vi "AutoRoutineSelector.vi"(6 "NotPurePursuit":bool, 8 "Routine":T1, 9 "OurSwitch":bool, 10 "OurScale":bool, 11 "Position":dbl) -> (3 "File Name":string)   [LabVIEW 2017]
uses:
  Shared/AutoRoutineSelector.ctl
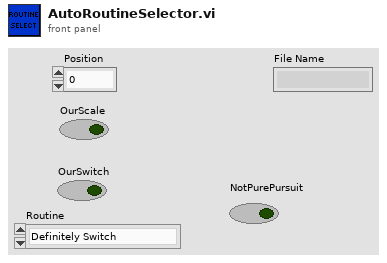
[diagram p1: front panel]
types:
  T1 = typedef "AutoRoutineSelector.ctl" = enum16{"Definitely Switch", "Definitely Scale", "Switch if in front, else scale", "Scale if in front, else switch", "Switch if in front, else cross line", "Scale if in front, else cross line", "Switch if in front, else scale if in front, else cross line ", "Scale if in front, else switch if in front, else cross line ", "Drive across line"}
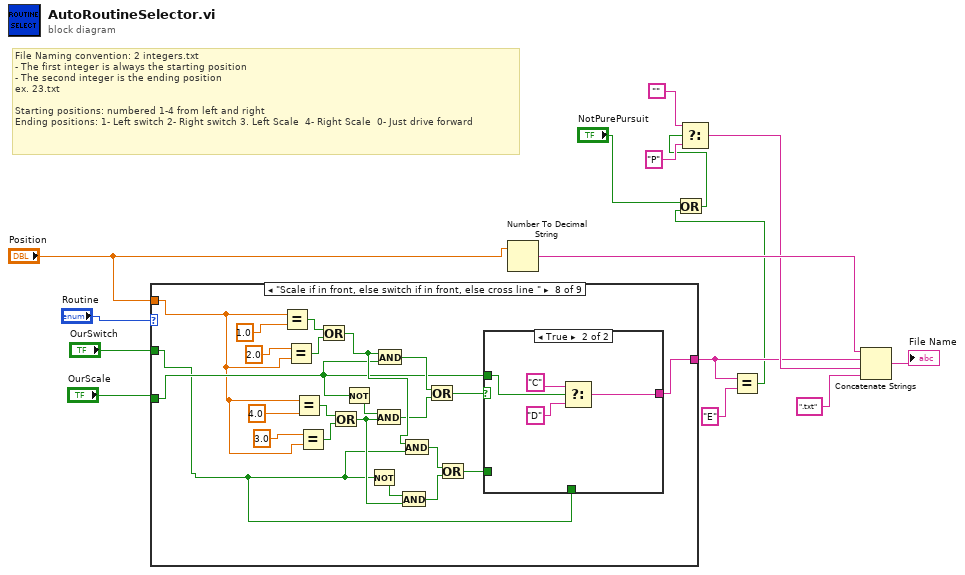
[diagram p0: block diagram]
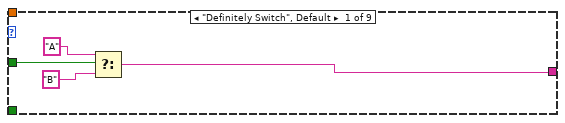
[diagram p2: hidden frame]
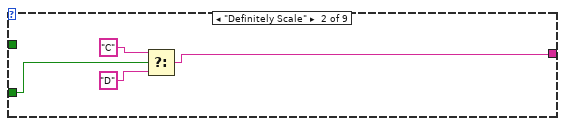
[diagram p3: hidden frame]
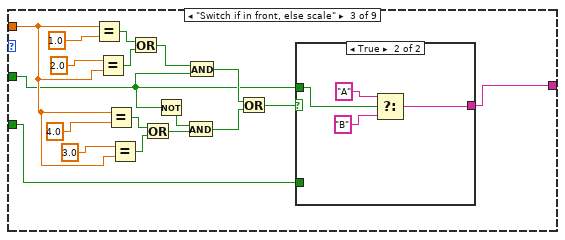
[diagram p4: hidden frame]
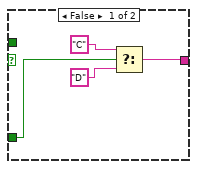
[diagram p5: hidden frame]
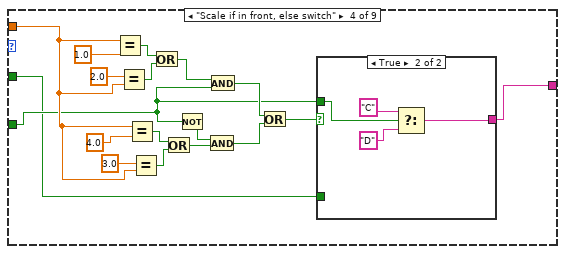
[diagram p6: hidden frame]
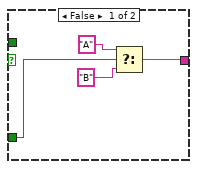
[diagram p7: hidden frame]
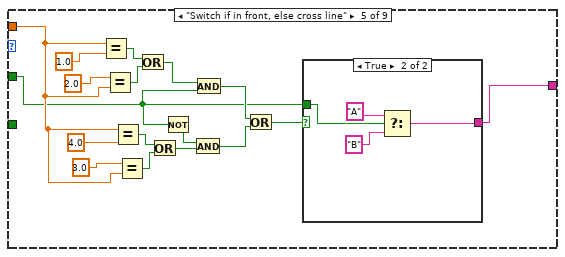
[diagram p8: hidden frame]
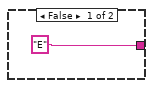
[diagram p9: hidden frame]
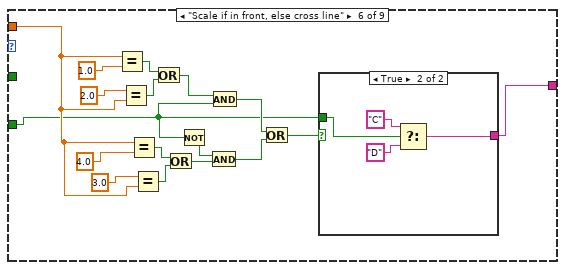
[diagram p10: hidden frame]
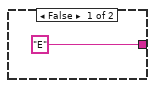
[diagram p11: hidden frame]
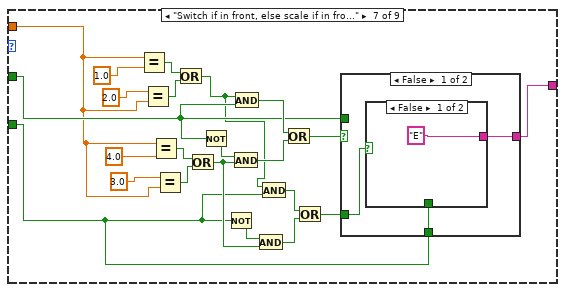
[diagram p12: hidden frame]
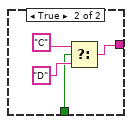
[diagram p13: hidden frame]
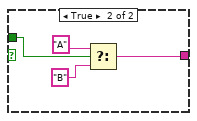
[diagram p14: hidden frame]
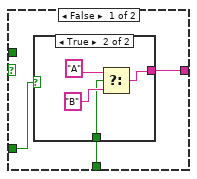
[diagram p15: hidden frame]
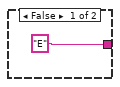
[diagram p16: hidden frame]
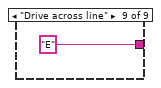
[diagram p17: hidden frame]
diagram:
  # "File Naming convention: 2 integers.txt \n- The first integer is always the starting position\n- The second integer is the ending position\nex. 23.txt\n\nStarting positions: numbered 1-4 from left and right\nEnding positions: 1- Left switch 2- Right switch 3. Left Scale  4- Right Scale  0- Just drive forward"
  n1 = case shown="\"Scale if in front, else switch if in front, else cross line \"" "Routine" {
    tunnel: "OurSwitch" -> [w19 _ w30 w55 w81 _ w129 w156 _]
    tunnel: "OurScale" -> [_ w23 w29 w56 _ w103 w120 w157 _]
    tunnel: [w16 w20 w24 w50 w76 w98 w127 w154 "E"] -> w4
    tunnel: "Position" -> [_ _ w36 w57 w82 w104 w128 w155 _]
    frame "Definitely Switch", Default {
      n2 = Select(t="A", s=w19, f="B") -> (s? t:f=w16:string)
    }
    frame "Definitely Scale" {
      n3 = Select(t="C", s=w23, f="D") -> (s? t:f=w20:string)
    }
    frame "Switch if in front, else scale" {
      n4 = Equal?(x=w36, y=1.0) -> (x = y?=w41:bool)
      n5 = Equal?(x=2.0 ("y"), y=w36) -> (x = y?=w40:bool)
      n6 = Equal?(x=w36, y=4.0) -> (x = y?=w37:bool)
      n7 = Equal?(x=3.0 ("y"), y=w36) -> (x = y?=w38:bool)
      n8 = Or(x=w41, y=w40) -> (x .or. y?=w39:bool)
      n9 = Or(x=w37, y=w38) -> (x .or. y?=w35:bool)
      n10 = Not(x=w30) -> (.not. x?=w34:bool)
      n11 = And(x=w34, y=w35) -> (x .and. y?=w32:bool)
      n12 = And(x=w39, y=w30) -> (x .and. y?=w33:bool)
      n13 = Or(x=w33, y=w32) -> (x .or. y?=w31:bool)
      n14 = case shown="True" w31 {
        tunnel: w30 -> [_ w49]
        tunnel: [w44 w46] -> w24
        tunnel: w29 -> [w45 _]
        frame False {
          n15 = Select(t="C", s=w45, f="D") -> (s? t:f=w44:string)
        }
        frame True {
          n16 = Select(t="A", s=w49, f="B") -> (s? t:f=w46:string)
        }
      }
    }
    frame "Scale if in front, else switch" {
      n17 = Equal?(x=w57, y=1.0) -> (x = y?=w58:bool)
      n18 = Equal?(x=2.0 ("y"), y=w57) -> (x = y?=w59:bool)
      n19 = Equal?(x=w57, y=4.0) -> (x = y?=w62:bool)
      n20 = Equal?(x=3.0 ("y"), y=w57) -> (x = y?=w61:bool)
      n21 = Or(x=w58, y=w59) -> (x .or. y?=w60:bool)
      n22 = Or(x=w62, y=w61) -> (x .or. y?=w63:bool)
      n23 = Not(x=w56) -> (.not. x?=w64:bool)
      n24 = And(x=w64, y=w63) -> (x .and. y?=w66:bool)
      n25 = And(x=w60, y=w56) -> (x .and. y?=w65:bool)
      n26 = Or(x=w65, y=w66) -> (x .or. y?=w67:bool)
      n27 = case shown="True" w67 {
        tunnel: w56 -> [_ w75]
        tunnel: [w70 w72] -> w50
        tunnel: w55 -> [w71 _]
        frame False {
          n28 = Select(t="A", s=w71, f="B") -> (s? t:f=w70:string)
        }
        frame True {
          n29 = Select(t="C", s=w75, f="D") -> (s? t:f=w72:string)
        }
      }
    }
    frame "Switch if in front, else cross line" {
      n30 = Equal?(x=w82, y=1.0) -> (x = y?=w83:bool)
      n31 = Equal?(x=2.0 ("y"), y=w82) -> (x = y?=w84:bool)
      n32 = Equal?(x=w82, y=4.0) -> (x = y?=w87:bool)
      n33 = Equal?(x=3.0 ("y"), y=w82) -> (x = y?=w86:bool)
      n34 = Or(x=w83, y=w84) -> (x .or. y?=w85:bool)
      n35 = Or(x=w87, y=w86) -> (x .or. y?=w88:bool)
      n36 = Not(x=w81) -> (.not. x?=w89:bool)
      n37 = And(x=w89, y=w88) -> (x .and. y?=w91:bool)
      n38 = And(x=w85, y=w81) -> (x .and. y?=w90:bool)
      n39 = Or(x=w90, y=w91) -> (x .or. y?=w92:bool)
      n40 = case shown="True" w92 {
        tunnel: w81 -> [_ w97]
        tunnel: ["E" w94] -> w76
        frame False {
        }
        frame True {
          n41 = Select(t="A", s=w97, f="B") -> (s? t:f=w94:string)
        }
      }
    }
    frame "Scale if in front, else cross line" {
      n42 = Equal?(x=w104, y=1.0) -> (x = y?=w114:bool)
      n43 = Equal?(x=2.0 ("y"), y=w104) -> (x = y?=w113:bool)
      n44 = Equal?(x=w104, y=4.0) -> (x = y?=w110:bool)
      n45 = Equal?(x=3.0 ("y"), y=w104) -> (x = y?=w111:bool)
      n46 = Or(x=w114, y=w113) -> (x .or. y?=w112:bool)
      n47 = Or(x=w110, y=w111) -> (x .or. y?=w109:bool)
      n48 = Not(x=w103) -> (.not. x?=w108:bool)
      n49 = And(x=w108, y=w109) -> (x .and. y?=w106:bool)
      n50 = And(x=w112, y=w103) -> (x .and. y?=w107:bool)
      n51 = Or(x=w107, y=w106) -> (x .or. y?=w105:bool)
      n52 = case shown="True" w105 {
        tunnel: w103 -> [_ w119]
        tunnel: ["E" w116] -> w98
        frame False {
        }
        frame True {
          n53 = Select(t="C", s=w119, f="D") -> (s? t:f=w116:string)
        }
      }
    }
    frame "Switch if in front, else scale if in front, else cross line " {
      n54 = Equal?(x=w128, y=1.0) -> (x = y?=w141:bool)
      n55 = Equal?(x=2.0 ("y"), y=w128) -> (x = y?=w140:bool)
      n56 = Equal?(x=w128, y=4.0) -> (x = y?=w138:bool)
      n57 = Equal?(x=3.0 ("y"), y=w128) -> (x = y?=w139:bool)
      n58 = Or(x=w141, y=w140) -> (x .or. y?=w124:bool)
      n59 = Or(x=w138, y=w139) -> (x .or. y?=w125:bool)
      n60 = Not(x=w129) -> (.not. x?=w137:bool)
      n61 = Not(x=w120) -> (.not. x?=w126:bool)
      n62 = And(x=w137, y=w125) -> (x .and. y?=w135:bool)
      n63 = And(x=w124, y=w129) -> (x .and. y?=w136:bool)
      n64 = And(x=w126, y=w125) -> (x .and. y?=w122:bool)
      n65 = And(x=w124, y=w120) -> (x .and. y?=w123:bool)
      n66 = Or(x=w136, y=w135) -> (x .or. y?=w134:bool)
      n67 = Or(x=w123, y=w122) -> (x .or. y?=w121:bool)
      n68 = case shown="False" w134 {
        tunnel: w129 -> [_ w153]
        tunnel: [w144 w150] -> w127
        tunnel: w121 -> [w143 _]
        tunnel: w120 -> [w142 _]
        frame False {
          n69 = case shown="False" w143 {
            tunnel: ["E" w147] -> w144
            tunnel: w142 -> [_ w146]
            frame False {
            }
            frame True {
              n70 = Select(t="C", s=w146, f="D") -> (s? t:f=w147:string)
            }
          }
        }
        frame True {
          n71 = Select(t="A", s=w153, f="B") -> (s? t:f=w150:string)
        }
      }
    }
    frame "Scale if in front, else switch if in front, else cross line " {
      n72 = Equal?(x=w155, y=1.0) -> (x = y?=w162:bool)
      n73 = Equal?(x=2.0 ("y"), y=w155) -> (x = y?=w163:bool)
      n74 = Equal?(x=w155, y=4.0) -> (x = y?=w165:bool)
      n75 = Equal?(x=3.0 ("y"), y=w155) -> (x = y?=w164:bool)
      n76 = Or(x=w162, y=w163) -> (x .or. y?=w172:bool)
      n77 = Or(x=w165, y=w164) -> (x .or. y?=w171:bool)
      n78 = Not(x=w157) -> (.not. x?=w166:bool)
      n79 = Not(x=w156) -> (.not. x?=w170:bool)
      n80 = And(x=w166, y=w171) -> (x .and. y?=w168:bool)
      n81 = And(x=w172, y=w157) -> (x .and. y?=w167:bool)
      n82 = And(x=w170, y=w171) -> (x .and. y?=w174:bool)
      n83 = And(x=w172, y=w156) -> (x .and. y?=w173:bool)
      n84 = Or(x=w167, y=w168) -> (x .or. y?=w169:bool)
      n85 = Or(x=w173, y=w174) -> (x .or. y?=w175:bool)
      n86 = case shown="True" w169 {
        tunnel: w157 -> [_ w187]
        tunnel: [w178 w184] -> w154
        tunnel: w175 -> [w177 _]
        tunnel: w156 -> [w176 _]
        frame False {
          n87 = case shown="True" w177 {
            tunnel: ["E" w181] -> w178
            tunnel: w176 -> [_ w180]
            frame False {
            }
            frame True {
              n88 = Select(t="A", s=w180, f="B") -> (s? t:f=w181:string)
            }
          }
        }
        frame True {
          n89 = Select(t="C", s=w187, f="D") -> (s? t:f=w184:string)
        }
      }
    }
    frame "Drive across line" {
    }
  }
  n90 = Number To Decimal String(number="Position") -> (decimal integer string=w13:string)  [unwired: 1 in]
  n91 = Equal?(x=w4, y="E") -> (x = y?=w2:bool)
  n92 = Or(x="NotPurePursuit", y=w2) -> (x .or. y?=w1:bool)
  n93 = Select(t="", s=w1, f="P") -> (s? t:f=w8:string)
  n94 = Concatenate Strings(w13, w4, w8, ".txt") -> (→"File Name":string)
